vi "Partial Clear of Row in Listbox.vi"(10 "Rows to Clear":i32[](array[numeric]), 11 "MulticolumnListbox in":refnum<vi>) -> ()   [LabVIEW 2018, in "EMS User Interface Actor.lvlib" / "EMS User Interface.lvclass"]
uses:
  EMS User Interface.lvclass
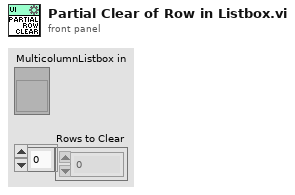
[diagram p1: front panel]
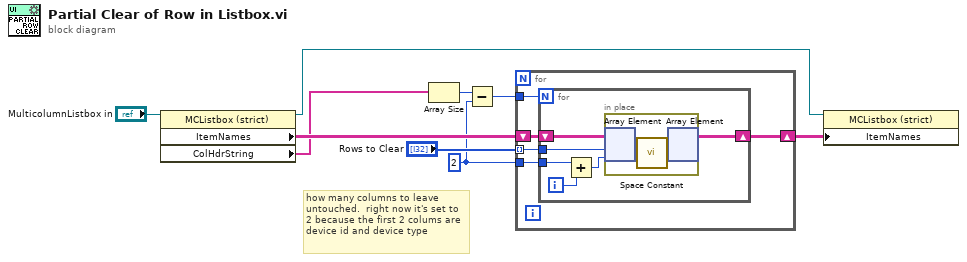
[diagram p0: block diagram]
diagram:
  w3 = 2 ("y")
  # "how many columns to leave untouched.  right now it's set to 2 because the first 2 colums are device id and device type"
  n1 = property class="MCListbox (strict)"(reference="MulticolumnListbox in") -> (reference out=w1:refnum<vi>, "ItemNames"=w7:string[][], "ColHdrString"=w6:string[])  [unwired: 1 in, 1 out]
  n2 = Array Size(array=w6) -> (size(s)=w5:i32)
  n3 = Subtract(x=w5, y=w3) -> (x-y=w4:i32)
  n4 = for {
    tunnel: "Rows to Clear" -> [w13] mode=indexing
    shift-right: [w12] -> w2
    shift-left: w7 -> [w14]
    tunnel: w4 -> [w11]
    tunnel: w3 -> [w10]
    n5 = for {
      N: w11 -> [_]
      tunnel: w13 -> [w19]
      shift-right: [w18] -> w12
      shift-left: w14 -> [w20]
      tunnel: w10 -> [w16]
      i -> [w17]
      n6 = Add(x=w16, y=w17) -> (x+y=w15:i32)
      n7 = in-place {
        n8 = in-place-array #1(w20, w19, w15) -> ()  [unwired: 1 out]
        n9 = call <vilib>:"Space Constant.vi"() -> ("String"=w21:string)
        n10 = in-place-array #1(w21) -> (w18:string[][])  [unwired: 2 out]
      }
    }
  }
  n11 = property class="MCListbox (strict)"(reference=w1, "ItemNames"=w2) -> ()  [unwired: 1 in, 2 out]
